vi "FTW-CodeGen-AdaptToInputs.vi"(0 "State In":T1={"Terminal Type"=variant(string ""), "PathWired"=FALSE}, 5 "XRef":refnum<vi>, 7 "Term Types":cluster{"Type":variant, "ID":string}[](array[cluster])) -> (4 "State Out":T1={"Terminal Type"=variant(string ""), "PathWired"=FALSE}, 6 "Reply":string[](array[string]))   [LabVIEW 2014, in "FTW-JSON-Fetch.xnode"]
uses:
  FTW-JSON-Fetch.xnode
  FTW-CodeGen-State.ctl
  FTW-CodeGen-XNodeReplyType.ctl
panel:
  # "Inputs"
  # "Outputs"
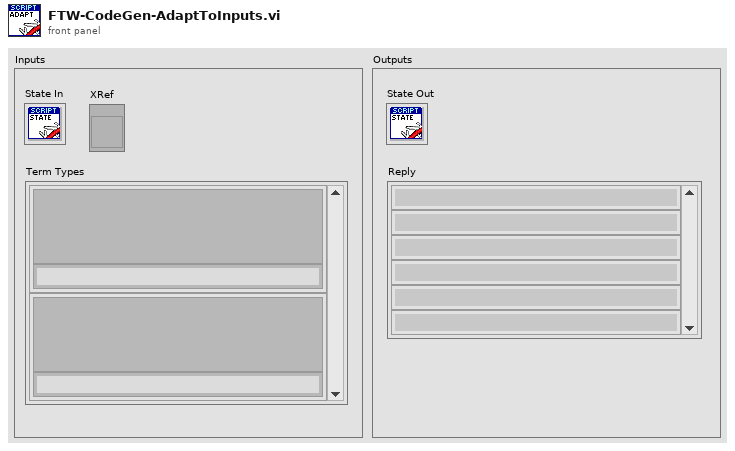
[diagram p1: front panel]
types:
  T1 = typedef "FTW-JSON-Fetch.xnode/FTW-CodeGen-State.ctl" = cluster{"Terminal Type":variant, "PathWired":bool}
  T2 = typedef "FTW-CodeGen-XNodeReplyType.ctl" = enum16{"UpdateState", "AdaptToInputs", "AdaptAndAugment", "CosmeticUpdate", "NoReply"}
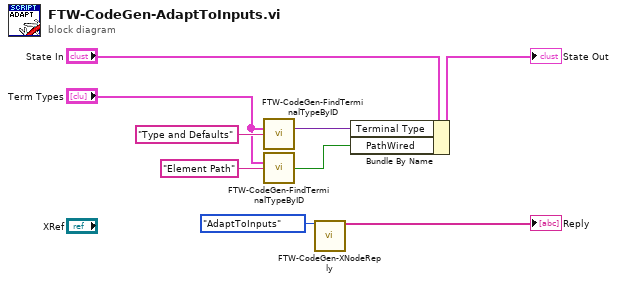
[diagram p0: block diagram]
diagram:
  n1 = call "FTW-CodeGen-FindTerminalTypeByID.vi"("Terminals"="Term Types", "Terminal ID"="Type and Defaults") -> ("Terminal Type"=w4:variant)  [unwired: 12 in, 1 out]
  n2 = call "FTW-CodeGen-FindTerminalTypeByID.vi"("Terminals"="Term Types", "Terminal ID"="Element Path") -> ("Found?"=w1:bool)  [unwired: 12 in, 1 out]
  n3 = call "FTW-CodeGen-XNodeReply.vi"("XNode Reply Type"=FTW-CodeGen-XNodeReplyType."AdaptToInputs") -> ("Reply"=→"Reply":string[])  [unwired: 14 in]
  n4 = Bundle By Name(cluster="State In", "Terminal Type"=w4, "PathWired"=w1) -> (→"State Out":T1)
